vi "RapidScan.vi"(0 "File Name?":string="temp", 1 "Scan Length (mm)":dbl=10.0 format="%.2f", 2 "Scan Len (mm) Ax2":dbl=10.0 format="%.2f", 3 "Number of pts\nAx 2":i32=11, 5 "Pressure Cal Parameters":T11={"Center Freq (MHz)"=0.0, "PRF (kHz)"=1.0, "Pulse window (us)"=0.0, "Hydrophone"=enum."PAL #1048", "booster amp?"=TRUE} {"Pulse window (us)" format="%.2f"; "PRF (kHz)" format="%.2f"; "Center Freq (MHz)" format="%.2f"}, 6 "Type of scan":u16(ring)=1 items=["Therapy With Scan", "M scan", "M Scan With Therapy Burst", "1-D B Scan", "1-D B Scan With Therapy Burst", "2-D B Scan", "2-D B Scan With Therapy Burst", "Rotational Scan", "1-D B-Scan PRF", "2-D B-Scan PRF", "Real-Time Scan", "Contrast Agents", "1-D w/ Real-Time Set Up", "Amplifier blah blah"], 7 "Therapy":bool, 8 "Digitizer Settings":T2={"Digitizer delay (us) "=0.0, "rf points per line"=2048, "lines per plane"=128, "Samp Rate (Hz)"=100000000.0, "Additional dig delay (us)"=0.0, "Voltage Scale"=0.4, "Pre-Looks"=0, "Offset delay (us)"=0.0, "bits A/D"=8, "Avg Num"=1, "DigTimeOut"=5.0, "Rel Dig Delay"=0.0, "Dig Ch"=0, "LeCroyCluster"={"LeCroy Channels"=[TRUE, FALSE, FALSE, FALSE], "LC read pt offset"=0.0, "Sweep Avg"=FALSE}, "Main Digitizer"=enum."NI Digitizer", "Dig Config"=enum."Single channel", "Digitizer ID Cluster"={"Acqiris/Alazar/SP ID"=[], "NI Instr Handles"=[], "LeCroy VISA"="", "GaGe Handle"={"Handle"=0, "Sample size"=0, "Resolution"=0, "Offset"=0, "Channels"=0, "Boards"=0}, "ATS Ref"="ATS9350", "Acqiris Address"=["PCI::INSTR0"], "ADQRef"=refnum, "adq_cu_ptr"=refnum}, "Trigger Settings"={"Trig Source"=1, "Trig Coupling"=0, "Trig Slope"=0, "Level (mV)"=1500.0}, "Bulk Acq"=FALSE, "Bulk Start Indexes"=[], "Data Ref RF"=refnum, "NI ID/Channel"=[], "Total Dig CH"=5, "Xtra Ann Trig delay (us)"=10.0, "Fix Z Delay?"=FALSE, "One Way Transmission?"=FALSE, "Data Ref Log"=refnum} {"Trigger Settings"."Trig Slope" items=["Positive", "Negative"]; "Trigger Settings"."Level (mV)" format="%.2f"; "Trigger Settings"."Trig Coupling" items=["DC 1 MOhm", "AC 1 MOhm", "DC 50 Ohm", "AC 50 Ohm"]; "Trigger Settings"."Trig Source" items=["Chan 1", "External"]; "Rel Dig Delay" format="%.2f"; "DigTimeOut" format="%.2f"; "Avg Num" min=1; "Offset delay (us)" format="%.2f"; "Additional dig delay (us)" format="%.2f"; "Digitizer delay (us)" format="%.2f"}, 9 "Motion Settings":T6={"No Motion?"=FALSE, "Motion System"=enum."No Motion Card", "Motion Bd ID"=1, "Motion Profile"="SMAC1", "# Axis"=1, "Reverse Z axis?"=TRUE, "SMAC Axis"=0, "scan pair"=enum."y-(x) scan", "RT fps"=6.0, "Steps per mm"=[1000, 1000, 1000, 1000], "Motor Parameters"={"velocity ct/s"=[10000.0, 10000.0, 10000.0, 50000.0], "accel ct/s^2"=[50000.0, 50000.0, 50000.0, 200000.0]}, "One Way Scan"=FALSE, "Reverse One Way Scan"=FALSE, "Global Position (mm)"=[], "Plane"=0, "Distance between\nscan lines (um)"=0.0, "Distance between\nscan planes (um)"=0.0, "number of scan planes"=1, "Total steps in line"=0, "Xtra plane\ndistance  (um)"=100, "Xtra planes "=1, "Add Axis"=FALSE, "overshoot cts"=200, "BKPT Shift"=0, "Scan Start Time (ms)"=0, "ESP VISA"="GPIB::1::INSTR", "3rd Axis"=1, "GL Ref Out"=refnum, "Galil Address"=""} {"3rd Axis" items=["x", "y", "z", "w"]; "Xtra planes" min=1; "Xtra plane\ndistance  (um)" min=0; "Distance between\nscan planes (um)" format="%.2f"; "Distance between\nscan lines (um)" format="%.2f"; "SMAC Axis" items=["None"=0, "Axis 1"=1, "Axis 2"=2, "Axis 3"=3, "Axis 4"=4, "Axis 5"=5, "Axis 6"=6, "Axis 7"=7, "Axis 8"=8, "Vector Space 1"=17, "Vector Space 2"=18, "Vector Space 3"=19, "Vector Space 4"=20]; "Motion Bd ID" min=1 max=32 step=1}) -> (14 "Scan data":T10 {"Pulse Parameters"."pos peak pressure (MPa)" format="%.2f"; "axis 2 ticks" format="%.2f"; "axis 1 ticks" format="%.2f"; "step size" format="%.2f"; "axis2o" format="%.2f"; "axis1o" format="%.2f"; "scan data" format="%.2f"}, 15 "Digitizer Settings Out":T2={"Digitizer delay (us) "=0.0, "rf points per line"=2048, "lines per plane"=128, "Samp Rate (Hz)"=100000000.0, "Additional dig delay (us)"=0.0, "Voltage Scale"=0.4, "Pre-Looks"=0, "Offset delay (us)"=0.0, "bits A/D"=8, "Avg Num"=1, "DigTimeOut"=5.0, "Rel Dig Delay"=0.0, "Dig Ch"=0, "LeCroyCluster"={"LeCroy Channels"=[TRUE, FALSE, FALSE, FALSE], "LC read pt offset"=0.0, "Sweep Avg"=FALSE}, "Main Digitizer"=enum."NI Digitizer", "Dig Config"=enum."Single channel", "Digitizer ID Cluster"={"Acqiris/Alazar/SP ID"=[], "NI Instr Handles"=[], "LeCroy VISA"="", "GaGe Handle"={"Handle"=0, "Sample size"=0, "Resolution"=0, "Offset"=0, "Channels"=0, "Boards"=0}, "ATS Ref"="ATS9350", "Acqiris Address"=["PCI::INSTR0"], "ADQRef"=refnum, "adq_cu_ptr"=refnum}, "Trigger Settings"={"Trig Source"=1, "Trig Coupling"=0, "Trig Slope"=0, "Level (mV)"=1500.0}, "Bulk Acq"=FALSE, "Bulk Start Indexes"=[], "Data Ref RF"=refnum, "NI ID/Channel"=[], "Total Dig CH"=5, "Xtra Ann Trig delay (us)"=10.0, "Fix Z Delay?"=FALSE, "One Way Transmission?"=FALSE, "Data Ref Log"=refnum} {"Trigger Settings"."Trig Slope" items=["Positive", "Negative"]; "Trigger Settings"."Level (mV)" format="%.2f"; "Trigger Settings"."Trig Coupling" items=["DC 1 MOhm", "AC 1 MOhm", "DC 50 Ohm", "AC 50 Ohm"]; "Trigger Settings"."Trig Source" items=["Chan 1", "External"]; "Rel Dig Delay" format="%.2f"; "DigTimeOut" format="%.2f"; "Avg Num" min=1; "Offset delay (us)" format="%.2f"; "Additional dig delay (us)" format="%.2f"; "Digitizer delay (us)" format="%.2f"}, 16 "Scan Params":T1={"File Name"="", "Keep?"=FALSE, "Synth Foc?"=FALSE, "Microscopy Scan Mode"=enum."Overview Scan"}, 18 "Motion Settings Out":T6={"No Motion?"=FALSE, "Motion System"=enum."NI 735x", "Motion Bd ID"=1, "Motion Profile"="SMAC1", "# Axis"=1, "Reverse Z axis?"=TRUE, "SMAC Axis"=0, "scan pair"=enum."y-(x) scan", "RT fps"=6.0, "Steps per mm"=[1000, 1000, 1000, 1000], "Motor Parameters"={"velocity ct/s"=[10000.0, 10000.0, 10000.0, 50000.0], "accel ct/s^2"=[50000.0, 50000.0, 50000.0, 200000.0]}, "One Way Scan"=FALSE, "Reverse One Way Scan"=FALSE, "Global Position (mm)"=[], "Plane"=0, "Distance between\nscan lines (um)"=0.0, "Distance between\nscan planes (um)"=0.0, "number of scan planes"=1, "Total steps in line"=0, "Xtra plane\ndistance  (um)"=100, "Xtra planes "=1, "Add Axis"=FALSE, "overshoot cts"=200, "BKPT Shift"=0, "Scan Start Time (ms)"=0, "ESP VISA"="GPIB::1::INSTR", "3rd Axis"=1, "GL Ref Out"=refnum, "Galil Address"=""} {"3rd Axis" items=["x", "y", "z", "w"]; "Xtra planes" min=1; "Xtra plane\ndistance  (um)" min=0; "Distance between\nscan planes (um)" format="%.2f"; "Distance between\nscan lines (um)" format="%.2f"; "SMAC Axis" items=["None"=0, "Axis 1"=1, "Axis 2"=2, "Axis 3"=3, "Axis 4"=4, "Axis 5"=5, "Axis 6"=6, "Axis 7"=7, "Axis 8"=8, "Vector Space 1"=17, "Vector Space 2"=18, "Vector Space 3"=19, "Vector Space 4"=20]; "Motion Bd ID" min=1 max=32 step=1}, 19 "Error Message":string)   [LabVIEW 2022 SP3]
uses:
  HydrophoneSettings.ctl
  Hydros.ctl
  ScanningControl/Digitizers/-DigitizerRoutines/DigitizerSettings.ctl
  ScanningControl/Digitizers/-DigitizerRoutines/Digitizer.ctl
  ScanningControl/Digitizers/-DigitizerRoutines/DigConfig.ctl
  ScanningControl/Digitizers/-DigitizerRoutines/DigitizerID.ctl
  C:/Windows/System32/ADQAPI_dotNet_helper.dll
  ScanningControl/Motion Controllers/NI_controller/-NI_MotionRoutines/MotionParameters.ctl
  ScanningControl/Motion Controllers/NI_controller/-NI_MotionRoutines/MotionSys.ctl
  ScanningControl/Motion Controllers/-MotionRoutines/ScanAxis.ctl
  ScanningControl/Motion Controllers/-MotionRoutines/3rdAxis.ctl
  ScanningControl/-ScanSystem/Controls/ScanParams.ctl
  ScanningControl/Motion Controllers/-MotionRoutines/MotionGlobals.vi
panel:
  # "1-D and 2-D B scan settings"
  # "1-D and 2-D B scan settings"
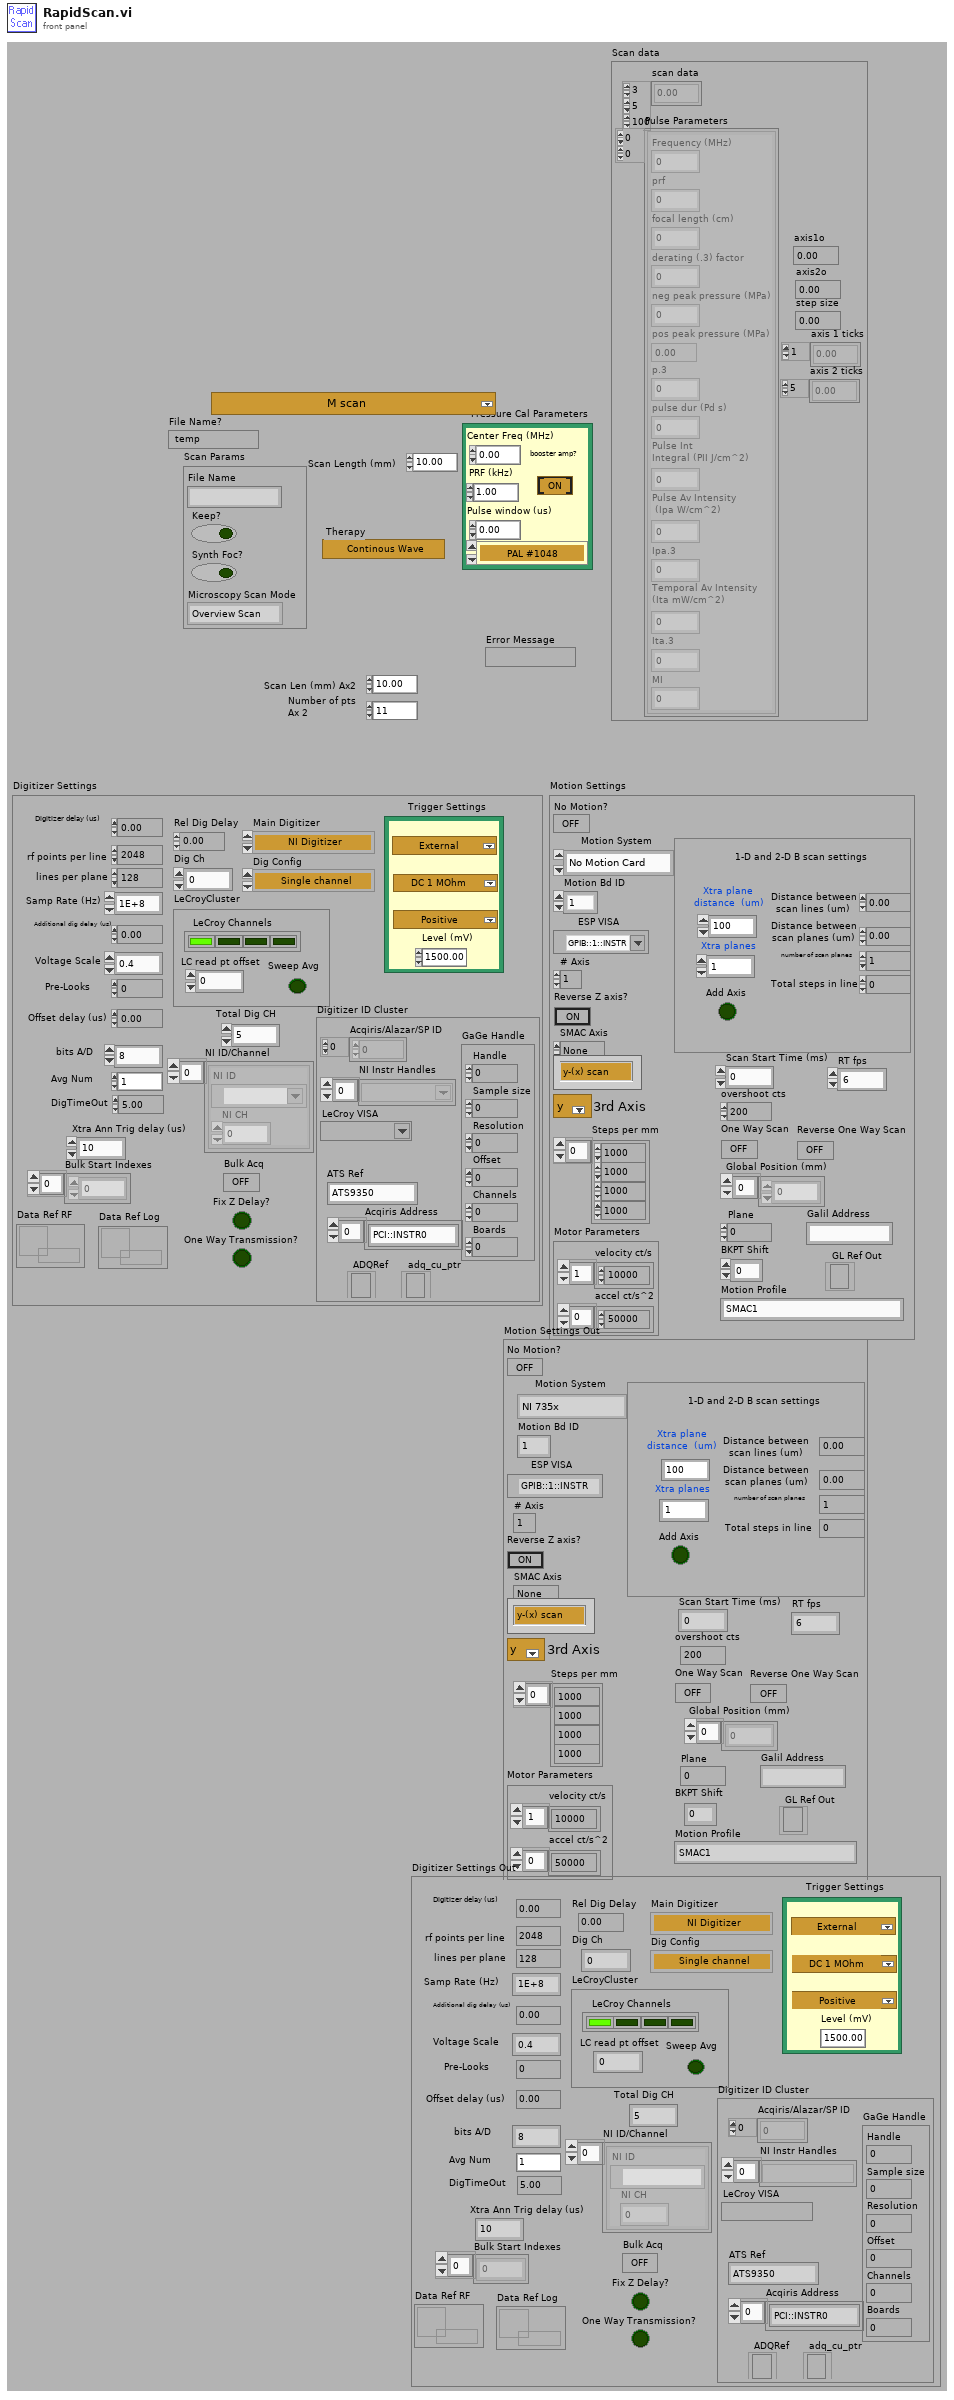
[diagram p1: front panel]
types:
  T1 = typedef "ScanParams.ctl" = cluster{"File Name":string, "Keep?":bool, "Synth Foc?":bool, "Microscopy Scan Mode":enum32{"Level X", "Level Y", "Overview Scan", "Detailed Scan", "V-Z Scan"}}
  T2 = typedef "DigitizerSettings.ctl" = cluster{"Digitizer delay (us) ":dbl, "rf points per line":i32, "lines per plane":i32, "Samp Rate (Hz)":dbl, "Additional dig delay (us)":dbl, "Voltage Scale":dbl, "Pre-Looks":i32, "Offset delay (us)":dbl, "bits A/D":i8, "Avg Num":i32, "DigTimeOut":sgl, "Rel Dig Delay":sgl, "Dig Ch":i32, "LeCroyCluster":cluster{"LeCroy Channels":bool[], "LC read pt offset":dbl, "Sweep Avg":bool}, "Main Digitizer":T3, "Dig Config":T4, "Digitizer ID Cluster":T5, "Trigger Settings":cluster{"Trig Source":u16, "Trig Coupling":u16, "Trig Slope":u16, "Level (mV)":dbl}, "Bulk Acq":bool, "Bulk Start Indexes":i32[], "Data Ref RF":refnum<data-value>, "NI ID/Channel":cluster{"NI ID":refnum<k15>, "NI CH":i32}[], "Total Dig CH":i32, "Xtra Ann Trig delay (us)":dbl, "Fix Z Delay?":bool, "One Way Transmission?":bool, "Data Ref Log":refnum<data-value>}
  T3 = typedef "Digitizer.ctl" = enum16{"Acqiris Digitizer", "NI Digitizer", "LeCroy", "GaGe", "AlazarTech", "No Digitizer", "Teledyne"}
  T4 = typedef "DigConfig.ctl" = enum16{"Single channel", "2 Chans w/ 2 Acqiris", "2 Chans w/ 1 Acqiris", "5-CH Pulser New", "5-CH pulser w/ ann array", "5-pass style ann array", "Empty"}
  T5 = typedef "DigitizerID.ctl" = cluster{"Acqiris/Alazar/SP ID":u32[], "NI Instr Handles":refnum<k15>[], "LeCroy VISA":refnum<visa-resource-name>, "GaGe Handle":cluster{"Handle":u32, "Sample size":u32, "Resolution":i32, "Offset":i32, "Channels":u32, "Boards":u32}, "ATS Ref":string, "Acqiris Address":string[], "ADQRef":refnum<k24>, "adq_cu_ptr":refnum<k24>}
  T6 = typedef "MotionParameters.ctl" = cluster{"No Motion?":bool, "Motion System":T7, "Motion Bd ID":u8, "Motion Profile":string, "# Axis":i8, "Reverse Z axis?":bool, "SMAC Axis":u16, "scan pair":T8, "RT fps":sgl, "Steps per mm":i32[], "Motor Parameters":cluster{"velocity ct/s":dbl[], "accel ct/s^2":dbl[]}, "One Way Scan":bool, "Reverse One Way Scan":bool, "Global Position (mm)":dbl[], "Plane":i32, "Distance between\nscan lines (um)":sgl, "Distance between\nscan planes (um)":sgl, "number of scan planes":i32, "Total steps in line":i32, "Xtra plane\ndistance  (um)":i32, "Xtra planes ":i32, "Add Axis":bool, "overshoot cts":i32, "BKPT Shift":i32, "Scan Start Time (ms)":u32, "ESP VISA":refnum<visa-resource-name>, "3rd Axis":T9, "GL Ref Out":refnum<k7>, "Galil Address":string}
  T7 = typedef "MotionSys.ctl" = enum16{"MM3000", "NI 735x", "Newport ESP", "No Motion Card", "Galil"}
  T8 = typedef "ScanAxis.ctl" = enum16{"y-(x) scan", "x-(y) scan", "z-(x) scan", "z-(y) scan", "y-(z) scan", "x-(z) scan", "w-(x) scan", "w-(y) scan", "w-(z) scan", "x-(w) scan", "y-(w) scan", "z-(w) scan"}
  T9 = typedef "3rdAxis.ctl" = u16
  T10 = cluster{"scan data":dbl[][][], "Pulse Parameters":cluster{"Frequency (MHz)":dbl, "prf":dbl, "focal length (cm)":dbl, "derating (.3) factor":dbl, "neg peak pressure (MPa)":dbl, "pos peak pressure (MPa)":dbl, "p.3":dbl, "pulse dur (Pd s)":dbl, "Pulse Int \nIntegral (PII J/cm^2)":dbl, "Pulse Av Intensity\n (Ipa W/cm^2)":dbl, "Ipa.3":dbl, "Temporal Av Intensity \n(Ita mW/cm^2)":dbl, "Ita.3":dbl, "MI":dbl}[][], "axis1o":dbl, "axis2o":dbl, "step size":dbl, "axis 1 ticks":dbl[], "axis 2 ticks":dbl[]}
  T11 = typedef "HydrophoneSettings.ctl" = cluster{"Center Freq (MHz)":dbl, "PRF (kHz)":dbl, "Pulse window (us)":dbl, "Hydrophone":T12, "booster amp?":bool}
  T12 = typedef "Hydros.ctl" = enum16{"PAL #1048", "PAL #525", "PAL #430a", "PAL #192", "DEAD PAL # 1403", "LOST UHI Onda", "DEAD PAL #1818", "PAL #1974", "DEAD #2266 w/booster", "PAL #2524 w/booster", "PAL FP21-20T", "PAL FP160-13  ", "PAL FP141-20", "PAL FP158-08T"}
  T13 = cluster{"Frequency (MHz)":dbl, "prf":dbl, "focal length (cm)":dbl, "derating (.3) factor":dbl, "neg peak pressure (MPa)":dbl, "pos peak pressure (MPa)":dbl, "p.3":dbl, "pulse dur (Pd s)":dbl, "Pulse Int \nIntegral (PII J/cm^2)":dbl, "Pulse Av Intensity\n (Ipa W/cm^2)":dbl, "Ipa.3":dbl, "Temporal Av Intensity \n(Ita mW/cm^2)":dbl, "Ita.3":dbl, "MI":dbl}[][]
  T14 = cluster{"Axis 1 Start":dbl, "Axis 2 Start":dbl, "Step Size":dbl, "Axis 1 Ticks":dbl[], "Axis 2 Ticks":dbl[]}
  T15 = cluster{dbl[][][], "Data":cluster{"Frequency (MHz)":dbl, "prf":dbl, "focal length (cm)":dbl, "derating (.3) factor":dbl, "neg peak pressure (MPa)":dbl, "pos peak pressure (MPa)":dbl, "p.3":dbl, "pulse dur (Pd s)":dbl, "Pulse Int \nIntegral (PII J/cm^2)":dbl, "Pulse Av Intensity\n (Ipa W/cm^2)":dbl, "Ipa.3":dbl, "Temporal Av Intensity \n(Ita mW/cm^2)":dbl, "Ita.3":dbl, "MI":dbl}[][], "Axis 1 Start":dbl, "Axis 2 Start":dbl, "Step Size":dbl, "Axis 1 Ticks":dbl[], "Axis 1 Ticks":dbl[]}
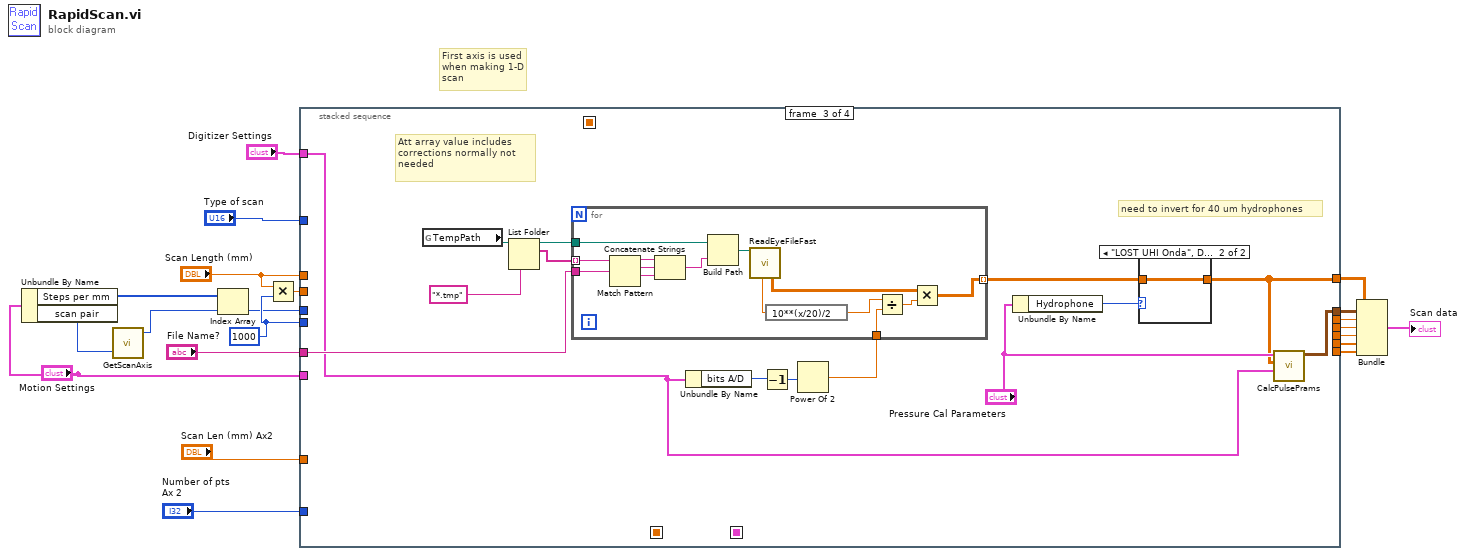
[diagram p0: block diagram]
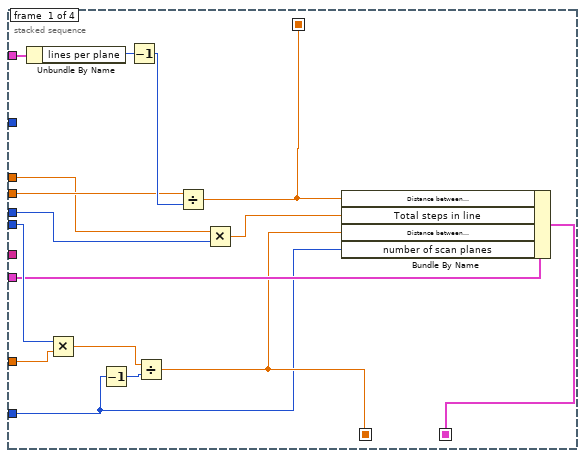
[diagram p2: hidden frame]
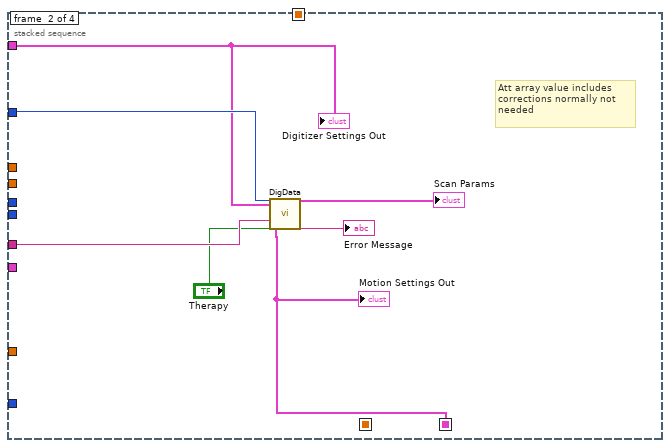
[diagram p3: hidden frame]
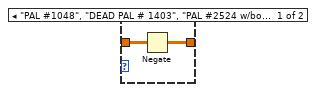
[diagram p4: hidden frame]
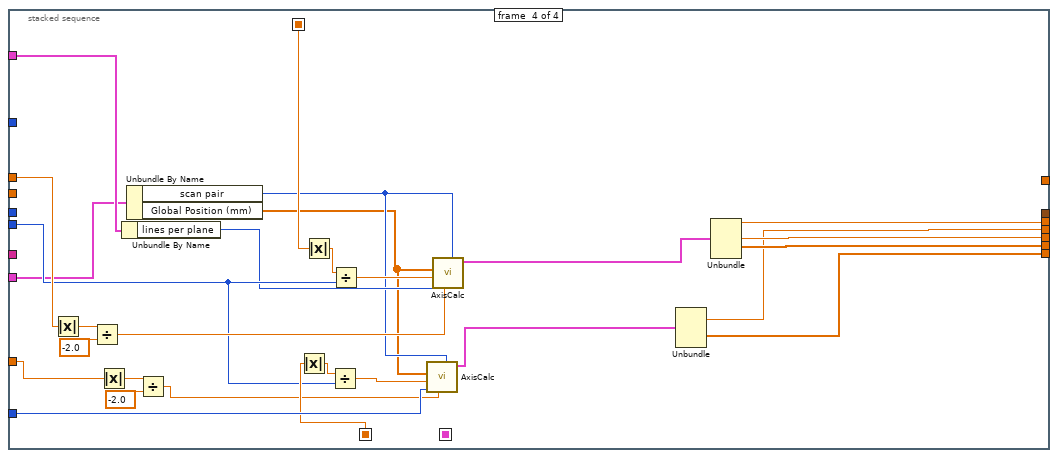
[diagram p5: hidden frame]
diagram:
  w2 = 1000
  # "First axis is used when making 1-D scan"
  n1 = Unbundle By Name("Motion Settings") -> ("Steps per mm"=w5:i32[], "scan pair"=w4:T8)
  n2 = call "GetScanAxis.vi"("scan pair"=w4) -> ("Axis 1"=w3:i32)  [unwired: 1 in, 2 out]
  n3 = Index Array(array=w5, index=w3) -> (element=w1:i32)
  n4 = Multiply(x="Scan Length (mm)", y=w2) -> (x*y=w13:dbl)
  n5 = stacked-sequence {
    seq-local: [w29 _ _ _] -> [_ _ _ w103]
    seq-local: [w28 _ _ _] -> [_ _ _ w87]
    seq-local: [w26 _ _ _] -> [_ w39 _ _]
    tunnel: [_ _ w45 _] -> w21
    tunnel: [_ _ w55 _] -> w20
    tunnel: [_ _ _ w95] -> w18
    tunnel: [_ _ _ w82] -> w17
    tunnel: [_ _ _ w94] -> w16
    tunnel: [_ _ _ w93] -> w15
    tunnel: [_ _ _ w81] -> w14
    tunnel: w13 -> [w25 _ _ _]
    tunnel: w2 -> [w35 _ _ w86]
    tunnel: "Type of scan" -> [_ w41 _ _]
    tunnel: "Scan Length (mm)" -> [w23 _ _ w101]
    tunnel: "File Name?" -> [_ w44 w53 _]
    tunnel: "Scan Len (mm) Ax2" -> [w34 _ _ w90]
    tunnel: "Number of pts\nAx 2" -> [w27 _ _ w89]
    tunnel: "Digitizer Settings" -> [w32 w40 w49 w80]
    tunnel: "Motion Settings" -> [w30 _ _ w78]
    tunnel: w1 -> [w24 _ _ _]
    frame #0 {
      n6 = Unbundle By Name(w32) -> ("lines per plane"=w31:i32)
      n7 = Multiply(x=w35, y=w34) -> (x*y=w33:dbl)
      n8 = Decrement(x=w27) -> (x-1=w36:i32)
      n9 = Decrement(x=w31) -> (x-1=w37:i32)
      n10 = Divide(x=w33, y=w36) -> (x/y=w28:dbl)
      n11 = Divide(x=w25, y=w37) -> (x/y=w29:dbl)
      n12 = Multiply(x=w23, y=w24) -> (x*y=w22:dbl)
      n13 = Bundle By Name(cluster=w30, "Distance between\nscan lines (um)"=w29, "Total steps in line"=w22, "Distance between\nscan planes (um)"=w28, "number of scan planes"=w27) -> (w26:T6)
    }
    frame #1 {
      # "Att array value includes corrections normally not needed"
      n14 = call "DigData.vi"("Type of scan"=w41, "Digitizer Settings"=w40, "File Name In"=w44, "Therapy (T)"="Therapy", "Motion Settings In"=w39) -> ("Scan Params"=→"Scan Params":T1, "Error Message"=→"Error Message":string)  [unwired: 11 in, 10 out]
      "Motion Settings Out" <- w39
      "Digitizer Settings Out" <- w40
    }
    frame #2 {
      # "need to invert for 40 um hydrophones"
      # "Att array value includes corrections normally not needed"
      n15 = global read "MotionGlobals.vi" "TempPath"() -> (w56:path)
      n16 = List Folder(path=w56, pattern="*.tmp") -> (path out=w58:path, filenames=w54:string[])  [unwired: 1 in, 3 out]
      n17 = Unbundle By Name(w49) -> ("bits A/D"=w51:i8)
      n18 = Decrement(x=w51) -> (x-1=w52:i8)
      n19 = Power Of 2(x=w52) -> (2^x=w50:dbl)
      n20 = for {
        tunnel: w54 -> [w70] mode=indexing
        tunnel: w58 -> [w75]
        tunnel: [w73] -> w46 mode=indexing
        tunnel: w53 -> [w69]
        tunnel: w50 -> [w64]
        n21 = Match Pattern(string=w70, regular expression=w69) -> (before substring=w68:string, match substring=w67:string, after substring=w66:string)  [unwired: 1 in, 1 out]
        n22 = Concatenate Strings(w68, w67, w66) -> (w65:string)
        n23 = Build Path(base path=w75, name or relative path=w65) -> (appended path=w72:path)
        n24 = call "ReadEyeFileFast.vi"("new file path"=w72) -> ("Digitizer (dB)"=w71:sgl, "2-D data array"=w74:sgl[][])  [unwired: 1 in, 16 out]
        n25 = expression code="10**(x/20)/2"(w71) -> (w62:sgl)
        n26 = Divide(x=w62, y=w64) -> (x/y=w63:dbl)
        n27 = Multiply(x=w74, y=w63) -> (x*y=w73:dbl[][])
      }
      n28 = Unbundle By Name("Pressure Cal Parameters") -> ("Hydrophone"=w47:T12)
      n29 = case shown="\"LOST UHI Onda\", Default" w47 {
        tunnel: w46 -> [w60 w61]
        tunnel: [w59 w61] -> w45
        frame "PAL #1048", "DEAD PAL # 1403", "PAL #2524 w/booster" {
          n30 = Negate(x=w60) -> (-x=w59:dbl[][][])
        }
        frame "LOST UHI Onda", Default {
        }
      }
      n31 = call "CalcPulsePrams.vi"("Digitizer Settings"=w49, "Array"=w45, "Pressure Cal Parameters"="Pressure Cal Parameters") -> ("Data"=w55:T13)  [unwired: 8 in]
    }
    frame #3 {
      n32 = Absolute Value(x=w101) -> (abs(x)=w99:dbl)
      n33 = Divide(x=w99, y=-2.0) -> (x/y=w98:dbl)
      n34 = Absolute Value(x=w90) -> (abs(x)=w91:dbl)
      n35 = Unbundle By Name(w80) -> ("lines per plane"=w79:i32)
      n36 = Unbundle By Name(w78) -> ("scan pair"=w77:T8, "Global Position (mm)"=w76:dbl[])
      n37 = Divide(x=w91, y=-2.0) -> (x/y=w84:dbl)
      n38 = Absolute Value(x=w87) -> (abs(x)=w88:dbl)
      n39 = Absolute Value(x=w103) -> (abs(x)=w100:dbl)
      n40 = Divide(x=w88, y=w86) -> (x/y=w85:dbl)
      n41 = Divide(x=w100, y=w86) -> (x/y=w97:dbl)
      n42 = call "AxisCalc.vi"("ScanAxis"=w77, "start"=w84, "Number of pts\nper scan"=w89, "increment"=w85, "Global Position (mm)"=w76) -> ("axis"=w83:T14)  [unwired: 2 in, 4 out]
      n43 = call "AxisCalc.vi"("ScanAxis"=w77, "start"=w98, "Number of pts\nper scan"=w79, "increment"=w97, "Global Position (mm)"=w76) -> ("axis"=w96:T14)  [unwired: 2 in, 4 out]
      n44 = Unbundle(w83) -> ("Axis 2 Start"=w82:dbl, "Axis 1 Ticks"=w81:dbl[])  [unwired: 3 out]
      n45 = Unbundle(w96) -> ("Axis 1 Start"=w95:dbl, "Step Size"=w94:dbl, "Axis 1 Ticks"=w93:dbl[])  [unwired: 2 out]
    }
  }
  n46 = Bundle(w21, "Data"=w20, "Axis 1 Start"=w18, "Axis 2 Start"=w17, "Step Size"=w16, "Axis 1 Ticks"=w15, "Axis 1 Ticks"=w14) -> (→"Scan data":T15)  [unwired: 1 out]
